vi "多参数控制命令.vi"(8 "Error in":errorcluster caption="Error in (no error)", 10 "控制命令":u16(ring)=1 items=["启动测量（全部）"=1, "初始化（清洗）"=10, "停止测量（全部）"=11, "校时"=13, "启动测量（单个传感器）"=19, "停止测量（单个传感器）"=20], 11 "站号":u16(ring)=10 items=["氨氮"=3, "水温"=9, "pH值"=10, "溶解氧"=11, "电导率"=12, "浊度"=13, "叶绿素a"=14, "藻密度"=15, "蓝绿藻"=16, "氧化还原电位"=17, "溶解氧%"=18, "盐度"=19]) -> (0 "error out":errorcluster)   [LabVIEW 2016, in "斯坦道原位多参数.lvlib"]
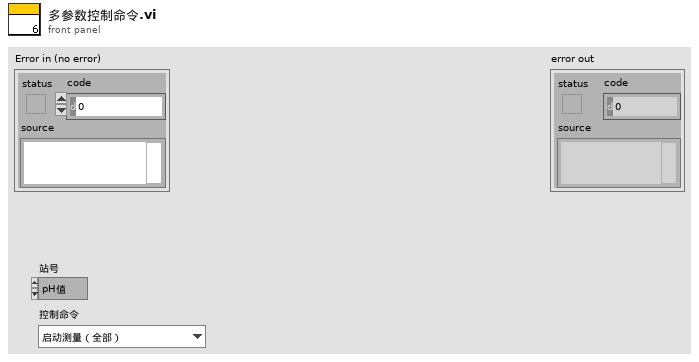
[diagram p1: front panel]
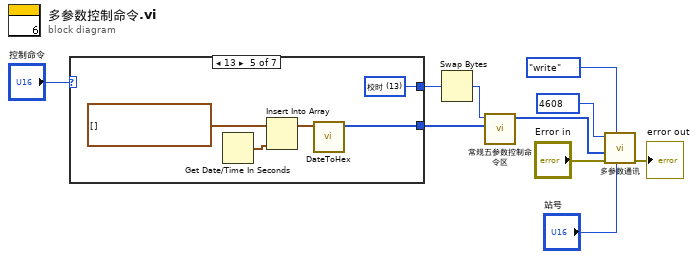
[diagram p0: block diagram]
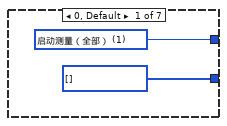
[diagram p2: hidden frame]
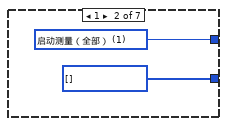
[diagram p3: hidden frame]
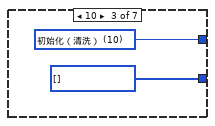
[diagram p4: hidden frame]
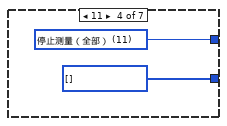
[diagram p5: hidden frame]
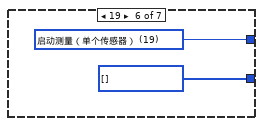
[diagram p6: hidden frame]
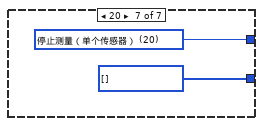
[diagram p7: hidden frame]
diagram:
  n1 = case shown="13" "控制命令" {
    tunnel: [u16[] [] ("控制命令参数") u16[] [] ("控制命令参数") u16[] [] ("控制命令参数") u16[] [] ("控制命令参数") w20 u16[] [] ("控制命令参数") u16[] [] ("控制命令参数")] -> w7
    tunnel: [w11 w13 w15 w17 w19 w25 w27] -> w6
    frame 0, Default {
      w11 = u16 1 items=["启动测量（全部）"=1, "初始化（清洗）"=10, "停止测量（全部）"=11, "校时"=13, "启动测量（单个传感器）"=19, "停止测量（单个传感器）"=20] ("控制命令")
    }
    frame 1 {
      w13 = u16 1 items=["启动测量（全部）"=1, "初始化（清洗）"=10, "停止测量（全部）"=11, "校时"=13, "启动测量（单个传感器）"=19, "停止测量（单个传感器）"=20] ("控制命令")
    }
    frame 10 {
      w15 = u16 10 items=["启动测量（全部）"=1, "初始化（清洗）"=10, "停止测量（全部）"=11, "校时"=13, "启动测量（单个传感器）"=19, "停止测量（单个传感器）"=20] ("控制命令")
    }
    frame 11 {
      w17 = u16 11 items=["启动测量（全部）"=1, "初始化（清洗）"=10, "停止测量（全部）"=11, "校时"=13, "启动测量（单个传感器）"=19, "停止测量（单个传感器）"=20] ("控制命令")
    }
    frame 13 {
      w19 = u16 13 items=["启动测量（全部）"=1, "初始化（清洗）"=10, "停止测量（全部）"=11, "校时"=13, "启动测量（单个传感器）"=19, "停止测量（单个传感器）"=20] ("控制命令")
      n2 = Get Date/Time In Seconds() -> (seconds since 1Jan1904=w23:timestamp)
      n3 = Insert Into Array(array=timestamp[] [] ("数组"), new element=w23) -> (w21:timestamp[])  [unwired: 1 in]
      n4 = call "DateToHex.vi"("DATE"=w21) -> ("数组"=w20:u16[])  [unwired: 10 in]
    }
    frame 19 {
      w25 = u16 19 items=["启动测量（全部）"=1, "初始化（清洗）"=10, "停止测量（全部）"=11, "校时"=13, "启动测量（单个传感器）"=19, "停止测量（单个传感器）"=20] ("控制命令")
    }
    frame 20 {
      w27 = u16 20 items=["启动测量（全部）"=1, "初始化（清洗）"=10, "停止测量（全部）"=11, "校时"=13, "启动测量（单个传感器）"=19, "停止测量（单个传感器）"=20] ("控制命令")
    }
  }
  n5 = Swap Bytes(anything=w6) -> (byte swapped=w5:u16)
  n6 = call "常规五参数控制命令区.vi"("控制命令参数"=w7, "控制命令"=w5) -> ("控制命令输出"=w3:u16[])  [unwired: 9 in]
  n7 = call "多参数通讯.vi"("Slave ID"="站号", "STEP"=enum16{"open", "read", "write", "close"}."write", "Error in"="Error in", "values"=w3, "starting address"=u16 4608) -> ("error out"=→"error out":errorcluster)  [unwired: 4 in, 2 out]
